vi "temperature_plotting2.vi"() -> ()   [LabVIEW 2021]
panel:
  out "XY Graph":cluster{i32[], dbl[]}(graph)
  out "Waveform Graph":dbl[][](graph)
  out "Waveform Chart":cluster{"Temperature (F)":dbl, "Celsius":dbl}(graph)
  in  "?":bool
  in  "On/Off":bool
  out "Temperature (F/C)":dbl(slide) scale=0.0..100.0
  in  "Temperature (F)":dbl(slide) scale=0.0..100.0
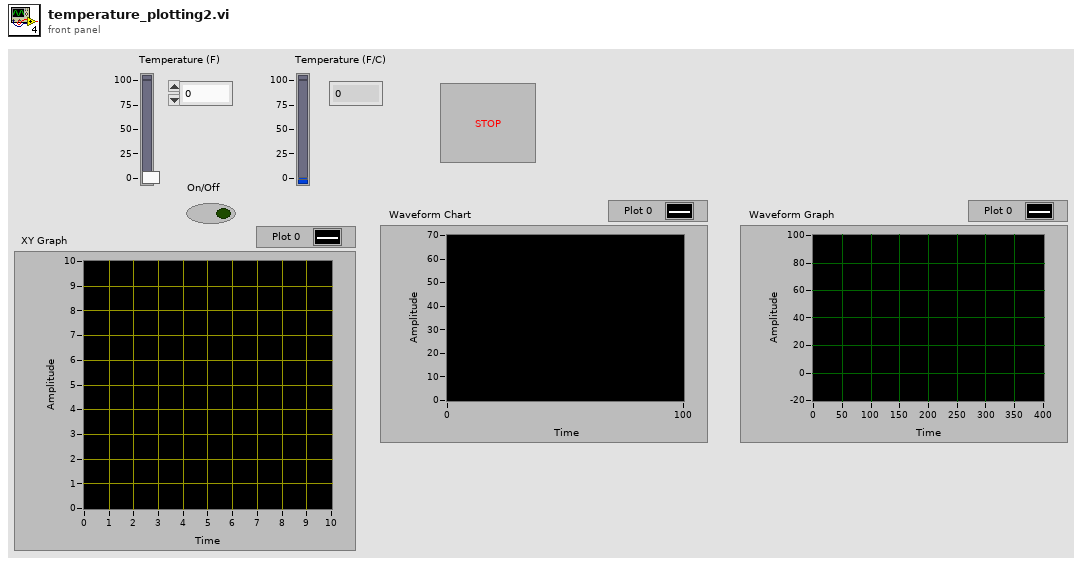
[diagram p1: front panel]
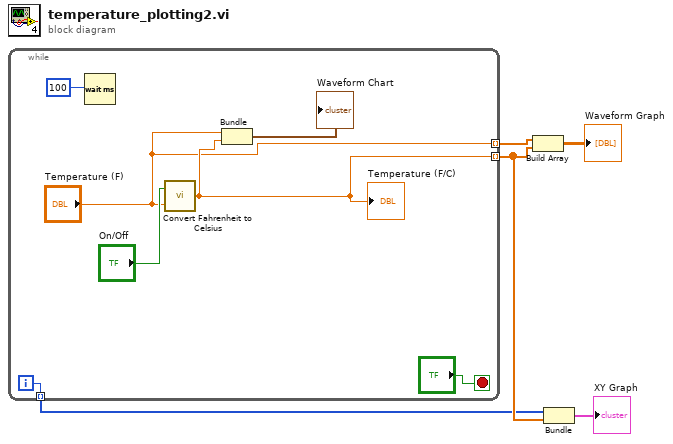
[diagram p0: block diagram]
diagram:
  n1 = while {
    tunnel: [w9] -> w3 mode=indexing
    tunnel: ["Temperature (F)"] -> w5 mode=indexing
    tunnel: [w6] -> w2 mode=indexing
    i -> [w6]
    stop <- "?" stop-if-true
    n2 = Wait (ms)(milliseconds to wait=100) -> ()  [unwired: 1 out]
    n3 = call "Convert Fahrenheit to Celsius.vi"("Fahrenheit"="Temperature (F)", "Boolean"="On/Off") -> ("Celsius"=w9:dbl)
    "Temperature (F/C)" <- w9
    n4 = Bundle("Temperature (F)"="Temperature (F)", "Celsius"=w9) -> (→"Waveform Chart":cluster{"Temperature (F)":dbl, "Celsius":dbl})  [unwired: 1 in]
  }
  n5 = Build Array(w5, w3) -> (→"Waveform Graph":dbl[][])
  n6 = Bundle(w2, w3) -> (→"XY Graph":cluster{i32[], dbl[]})  [unwired: 1 in]
